vi "Open FITS Reference.vi"(8 "error in (no error)":errorcluster, 11 "Save Image in":refnum<class "Save Image.lvclass">) -> (0 "error out":errorcluster, 3 "Save Image out":refnum<class "Save Image.lvclass">)   [LabVIEW 2018, in "Save Image.lvclass"]
uses:
  Save Image.lvclass
  Save Image.lvclass/Save Image.ctl
  <userlib>/gfitsio/gfitsio.lvlib
  Simulated_Header/Simulated_Header.lvclass
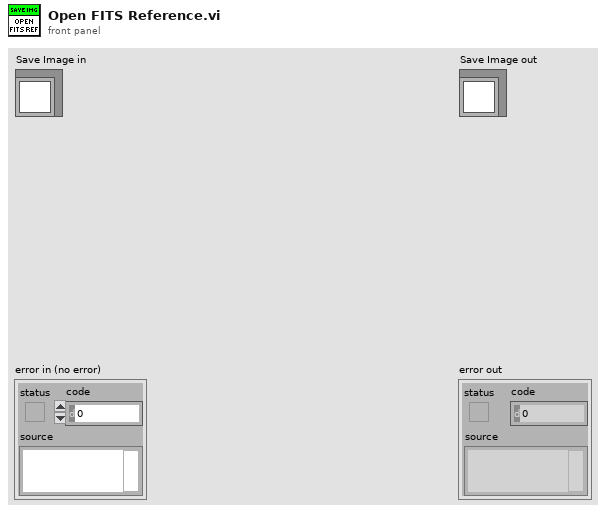
[diagram p1: front panel]
types:
  T1 = enum16{"open", "open or create", "create or replace", "create", "open (read only)"}
  T2 = cluster{"COMNENT":string, "OBSTYPE":string, "ACSVRSN":string, "CHANNEL":u16, "LAST_IMG_NAME":string, "NIGHTDIR":string}
  T3 = typedef "gfitsio.lvlib/gfitsio-refnum.ctl" = refnum<k1>
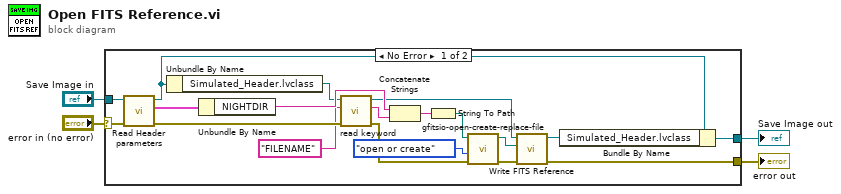
[diagram p0: block diagram]
diagram:
  n1 = case shown="No Error" "error in (no error)" {
    selector: "error in (no error)" -> [w21 w25]
    tunnel: [w18 w25] -> w3
    tunnel: [w15 w24] -> w1
    tunnel: "Save Image in" -> [w22 w24]
    frame No Error {
      n2 = call "Read Header parameters.vi"("error in (no error)"=w21, "Save Image in"=w22) -> ("error out"=w9:errorcluster, "Header parameters"=w14:T2, "Save Image out"=w16:refnum<class "Save Image.lvclass">)  [unwired: 7 in]
      n3 = Unbundle By Name(w16) -> ("Simulated_Header.lvclass"=w10:refnum<class "Simulated_Header.lvclass">)
      n4 = Unbundle By Name(w14) -> ("NIGHTDIR"=w13:string)
      n5 = call "read keyword.vi"("error in (no error)"=w9, "keyword"="FILENAME", "Simulated_Header in"=w10) -> ("error out"=w8:errorcluster, "value"=w5:string, "Simulated_Header out"=w7:refnum<class "Simulated_Header.lvclass">)  [unwired: 6 in]
      n6 = Concatenate Strings(w13, w5) -> (w12:string)
      n7 = String To Path(string=w12) -> (path=w11:path)
      n8 = call <userlib>:"gfitsio-open-create-replace-file.vi"("error in (no error)"=w8, "function (open)"=T1."open or create", "file path (dialog if empty)"=w11) -> ("error out"=w19:errorcluster, "gfits refnum"=w20:T3)  [unwired: 6 in, 1 out]
      n9 = call "Write FITS Reference.vi"("error in (no error)"=w19, "gfits refnum"=w20, "Simulated_Header in"=w7) -> ("error out"=w18:errorcluster, "Simulated_Header out"=w17:refnum<class "Simulated_Header.lvclass">)  [unwired: 7 in]
      n10 = Bundle By Name(cluster=w16, "Simulated_Header.lvclass"=w17) -> (w15:refnum<class "Save Image.lvclass">)
    }
    frame Error {
    }
  }
  "error out" <- w3
  "Save Image out" <- w1
